vi "CREATE EMAIL.vi"(9 "DATA IN":T2, 10 "BYU ID # IN":string, 11 "connection reference in":T3) -> (1 "SEND EMAIL":bool=TRUE, 2 "MESSAGE OUT":string, 3 "connection reference out":T3, 5 "USER EMAIL OUT":string)   [LabVIEW 2019]
uses:
  <vilib>/addons/database/Connection.llb/Conn ObjectReference.ctl
  Controls/Table Data Types/Inventory Data Type.ctl
  Controls/Table Data Types/User Data Type.ctl
  <vilib>/addons/database/_DB Variant To Data/Database Variant To Data.xnode
  <vilib>/addons/database/NI_Database_API.lvlib
panel:
  out "DATA OUT":T2
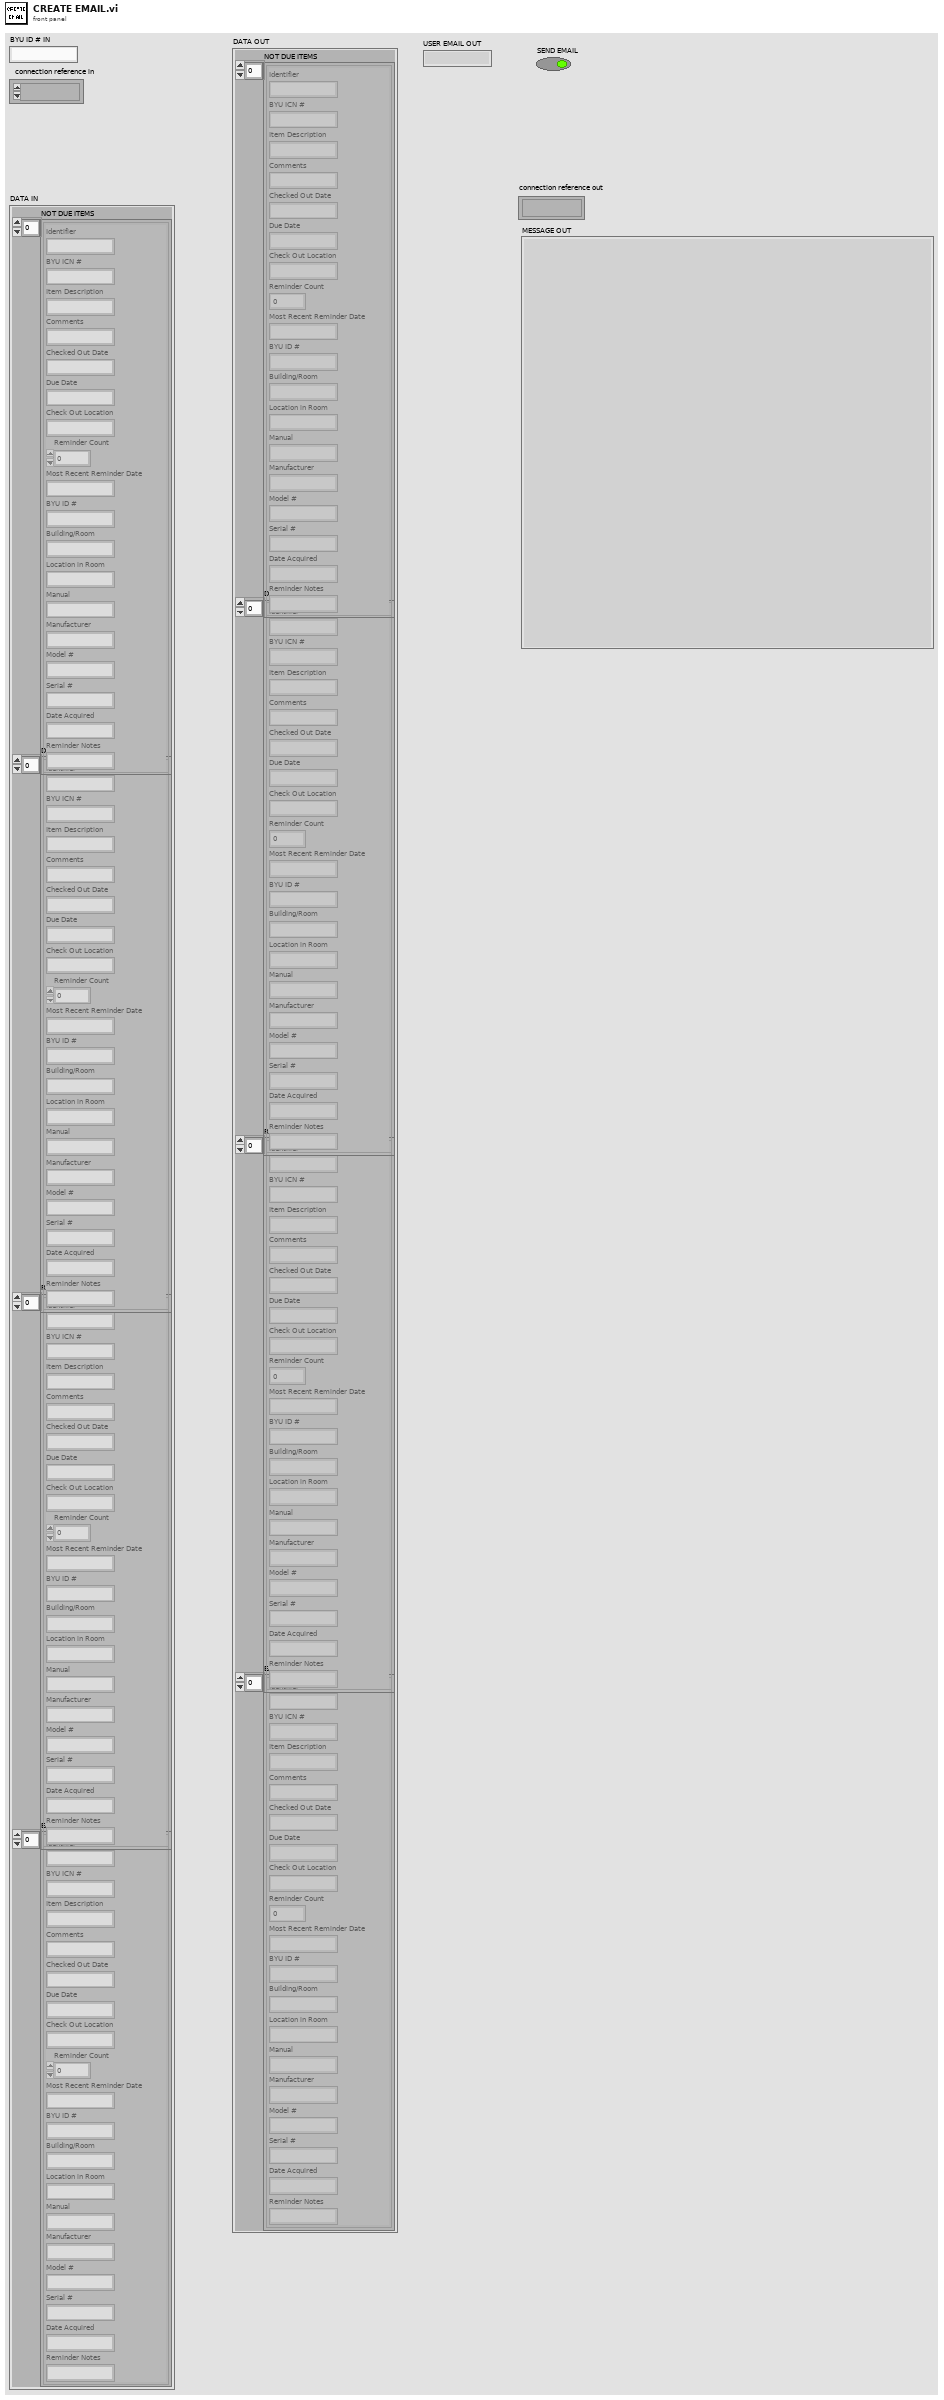
[diagram p1: front panel]
types:
  T1 = typedef "Inventory Data Type.ctl" = cluster{"Identifier":string, "BYU ICN #":string, "Item Description":string, "Comments":string, "Checked Out Date":string, "Due Date":string, "Check Out Location":string, "Reminder Count":i32, "Most Recent Reminder Date":string, "BYU ID #":string, "Building/Room":string, "Location in Room":string, "Manual":string, "Manufacturer":string, "Model #":string, "Serial #":string, "Date Acquired":string, "Reminder Notes":string}
  T2 = cluster{"NOT DUE ITEMS":T1[], "DUE ITEMS":T1[], "REMINDER ITEMS":T1[], "EARLY REMINDER ITEMS":T1[]}
  T3 = typedef "NI_Database_API.lvlib/Conn ObjectReference.ctl" = refnum<k1>
  T4 = typedef "User Data Type.ctl" = cluster{"BYU ID #":string, "First Name":string, "Last Name":string, "Phone Number":string, "Email":string, "Department":string, "Graduation Status":string, "Anticipated Graduation Year":string, "Credit Score":dbl, "Date Added":string, "Graduation Clearance Date":string, "Picture File Name":string, "User Comments":string}
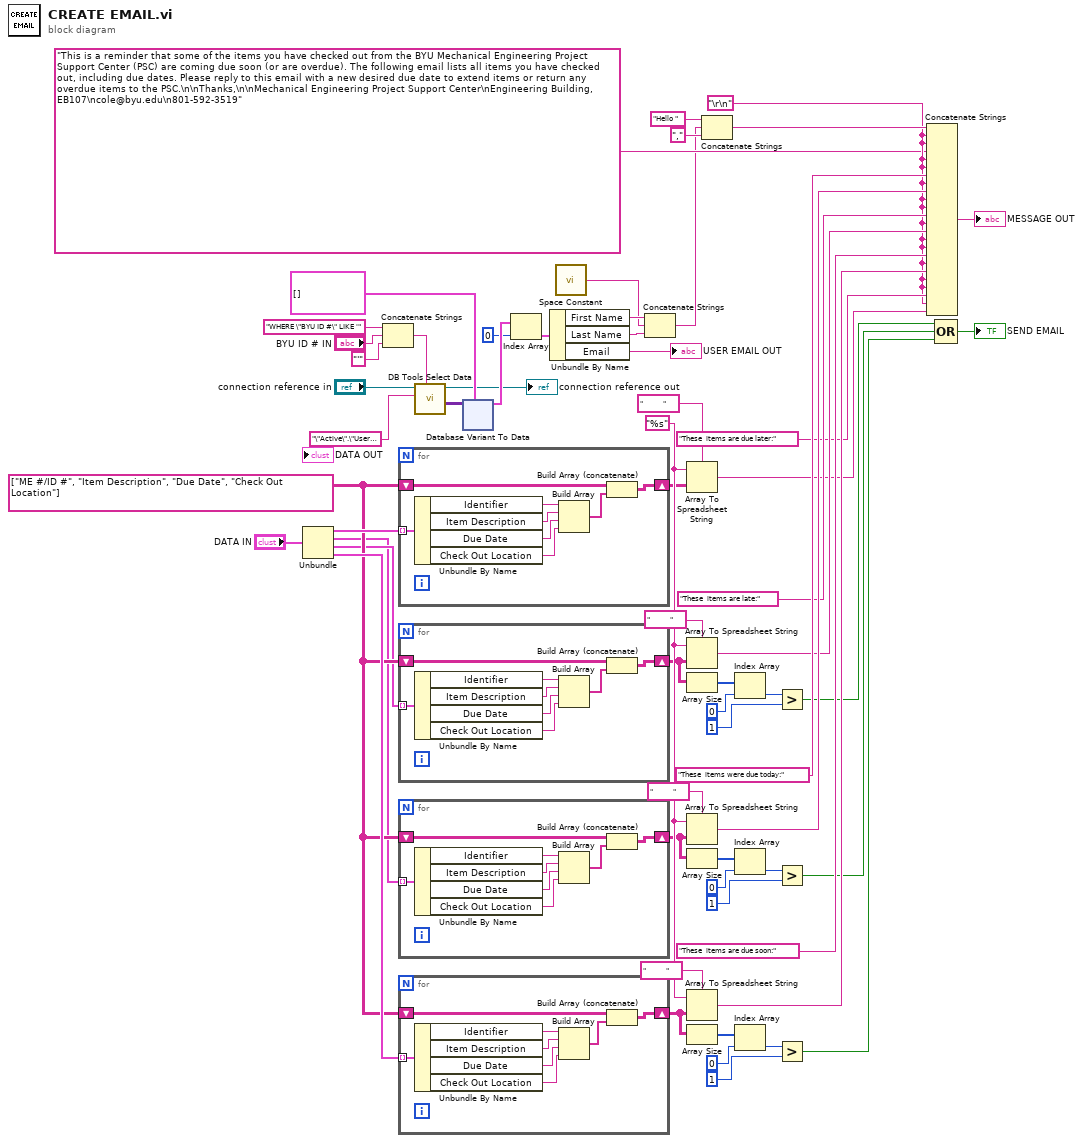
[diagram p0: block diagram]
diagram:
  w33 = "%s" ("table")
  w36 = "\r\n"
  w45 = string[][] [["ME #/ID #", "Item Description", "Due Date", "Check Out Location"]]
  n1 = Unbundle("DATA IN") -> ("NOT DUE ITEMS"=w47:T1[], "DUE ITEMS"=w5:T1[], "REMINDER ITEMS"=w6:T1[], "EARLY REMINDER ITEMS"=w46:T1[])
  n2 = Concatenate Strings("WHERE \"BYU ID #\" LIKE '" ("table"), "BYU ID # IN", "'" ("table")) -> (w57:string)
  n3 = for {
    tunnel: w47 -> [w70] mode=indexing
    shift-right: [w63] -> w32
    shift-left: w45 -> [w65]
    n4 = Unbundle By Name(w70) -> ("Identifier"=w69:string, "Item Description"=w68:string, "Due Date"=w67:string, "Check Out Location"=w66:string)
    n5 = Build Array(w69, w68, w67, w66) -> (w64:string[])
    n6 = Build Array (concatenate)(w65, w64) -> (w63:string[][])
  }
  n7 = for {
    tunnel: w6 -> [w78] mode=indexing
    shift-right: [w71] -> w31
    shift-left: w45 -> [w73]
    n8 = Unbundle By Name(w78) -> ("Identifier"=w77:string, "Item Description"=w76:string, "Due Date"=w75:string, "Check Out Location"=w74:string)
    n9 = Build Array(w77, w76, w75, w74) -> (w72:string[])
    n10 = Build Array (concatenate)(w73, w72) -> (w71:string[][])
  }
  n11 = for {
    tunnel: w5 -> [w86] mode=indexing
    shift-right: [w79] -> w30
    shift-left: w45 -> [w81]
    n12 = Unbundle By Name(w86) -> ("Identifier"=w85:string, "Item Description"=w84:string, "Due Date"=w83:string, "Check Out Location"=w82:string)
    n13 = Build Array(w85, w84, w83, w82) -> (w80:string[])
    n14 = Build Array (concatenate)(w81, w80) -> (w79:string[][])
  }
  n15 = for {
    tunnel: w46 -> [w94] mode=indexing
    shift-right: [w87] -> w29
    shift-left: w45 -> [w89]
    n16 = Unbundle By Name(w94) -> ("Identifier"=w93:string, "Item Description"=w92:string, "Due Date"=w91:string, "Check Out Location"=w90:string)
    n17 = Build Array(w93, w92, w91, w90) -> (w88:string[])
    n18 = Build Array (concatenate)(w89, w88) -> (w87:string[][])
  }
  n19 = call <vilib>:"DB Tools Select Data.vi"("condition"=w57, "table"="\"Active\".\"Users\"", "connection reference"="connection reference in") -> ("data"=w56:variant[][], "connection reference out"=→"connection reference out":T3)  [unwired: 3 in, 1 out]
  n20 = xnode "Database Variant To Data"("database variant"=w56, "type"=T4[] [] ("Array")) -> ("data"=w54:T4[])  [unwired: 1 in, 1 out]
  n21 = Index Array(array=w54, index=0) -> (element=w52:T4)
  n22 = Unbundle By Name(w52) -> ("First Name"=w4:string, "Last Name"=w3:string, "Email"=→"USER EMAIL OUT":string)
  n23 = call <vilib>:"Space Constant.vi"() -> ("String"=w2:string)
  n24 = Concatenate Strings(w4, w2, w3) -> (w1:string)
  n25 = Array To Spreadsheet String(delimiter (Tab)="          ", array=w32, 3:w33) -> (spreadsheet string=w35:string)
  n26 = Array To Spreadsheet String(delimiter (Tab)="          ", array=w31, 3:w33) -> (spreadsheet string=w40:string)
  n27 = Array Size(array=w31) -> (size(s)=w28:i32[])
  n28 = Array To Spreadsheet String(delimiter (Tab)="          ", array=w30, 3:w33) -> (spreadsheet string=w42:string)
  n29 = Array Size(array=w30) -> (size(s)=w27:i32[])
  n30 = Array To Spreadsheet String(delimiter (Tab)="          ", array=w29, 3:w33) -> (spreadsheet string=w38:string)
  n31 = Array Size(array=w29) -> (size(s)=w26:i32[])
  n32 = Concatenate Strings("Hello " ("table"), w1, "," ("table")) -> (w44:string)
  n33 = Index Array(array=w28, index=0) -> (element=w22:i32)
  n34 = Index Array(array=w27, index=0) -> (element=w20:i32)
  n35 = Index Array(array=w26, index=0) -> (element=w18:i32)
  n36 = Greater?(x=w22, y=1 ("index")) -> (0:w16:bool)
  n37 = Greater?(x=w20, y=1 ("index")) -> (0:w15:bool)
  n38 = Greater?(x=w18, y=1 ("index")) -> (0:w14:bool)
  n39 = Concatenate Strings(w44, w36, w36, "This is a reminder that some of the items you have checked out from the BYU Mechanical Engineering Project Support Center (PSC) are coming due soon (or are overdue). The following email lists all items you have checked out, including due dates. Please reply to this email with a new desired due date to extend items or return any overdue items to the PSC.\n\nThanks,\n\nMechanical Engineering Project Support Center\nEngineering Building, EB107\ncole@byu.edu\n801-592-3519" ("table"), w36, w36, "These  items were due today:" ("table"), w36, w42, w36, w36, "These  items are late:" ("table"), w36, w40, w36, w36, "These  items are due soon:" ("table"), w36, w38, w36, w36, "These  items are due later:" ("table"), w36, w35) -> (→"MESSAGE OUT":string)
  n40 = Compound Arithmetic op=OR(w16, w15, w14) -> (→"SEND EMAIL":bool)
